vi "Color Manipulation.vi"() -> ()   [LabVIEW 2014]
doc: "Use this template to build a VI to use as a subVI."
uses:
  <vilib>/vision/NI_Vision_Development_Module.lvlib
panel:
  out "Dst":T1(plugin-control)
  out "Src":T1(plugin-control)
  # ":: MVi Framework V1.0 ::\nAuthor:Gaoke Yang\nEmail: gaoke.yang@yahoo.com\nWeb: www.mvicontrol.com\nCopyright (C) 2015, MVI Technologies All Rights Reserved"
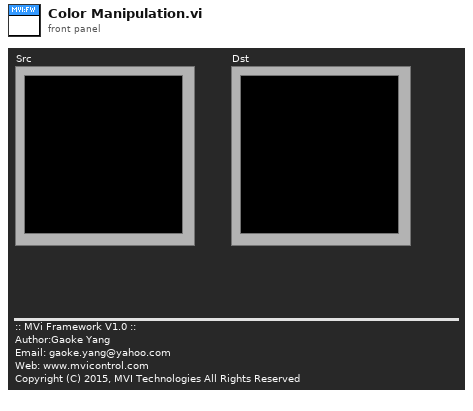
[diagram p1: front panel]
types:
  T1 = typedef "IMAQ Image.ctl" = refnum<image>
  T2 = typedef "Image Type" = u32
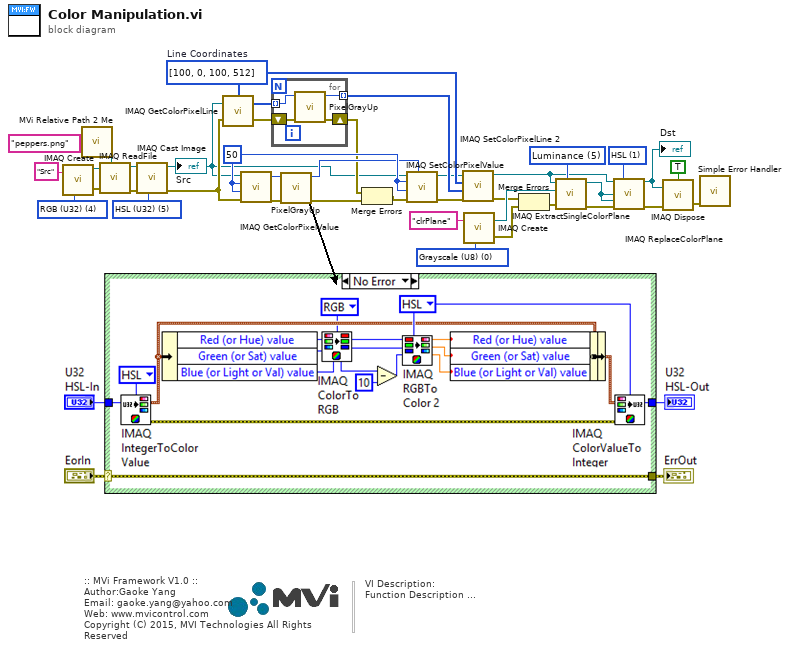
[diagram p0: block diagram]
diagram:
  w8 = u16 1 items=["RGB", "HSL", "HSV", "HSI"] ("Color Mode")
  w19 = 50 ("index")
  w21 = i32[] [100, 0, 100, 512]  # Line Coordinates
  w27 = T2 0 items=["Grayscale (U8)", "Grayscale (I16)", "Grayscale (SGL)", "Complex (CSG)", "RGB (U32)", "HSL (U32)", "RGB (U64)", "Grayscale (U16)"] ("Image Type")
  w28 = 5 items=["Red", "Green", "Blue", "Hue", "Saturation", "Luminance", "Value", "Intensity"] ("Color Plane")
  w29 = T2 4 items=["Grayscale (U8)", "Grayscale (I16)", "Grayscale (SGL)", "Complex (CSG)", "RGB (U32)", "HSL (U32)", "RGB (U64)", "Grayscale (U16)"] ("Image Type")
  w30 = T2 5 items=["Grayscale (U8)", "Grayscale (I16)", "Grayscale (SGL)", "Complex (CSG)", "RGB (U32)", "HSL (U32)", "RGB (U64)", "Grayscale (U16)"] ("Image Type")
  # "VI Description:\nFunction Description ..."
  # ":: MVi Framework V1.0 ::\nAuthor:Gaoke Yang\nEmail: gaoke.yang@yahoo.com\nWeb: www.mvicontrol.com\nCopyright (C) 2015, MVI Technologies All Rights Reserved"
  n1 = call "IMAQ Create"("Image Name"="Src" ("name or relative path"), "Image Type"=w29) -> ("New Image"=w34:T1, "error out"=w33:errorcluster)  [unwired: 2 in, 1 out]
  n2 = call "MVi Relative Path 2 Me.vi"("Relative Path"="peppers.png" ("name or relative path")) -> ("Appended Dir"=w35:path)  [unwired: 5 in, 1 out]
  n3 = call "IMAQ ReadFile"("File Path"=w35, "error in (no error)"=w33, "Image"=w34) -> ("error out"=w32:errorcluster, "Image Out"=w31:T1)  [unwired: 4 in, 3 out]
  n4 = call "IMAQ Cast Image"("Image Type"=w30, "error in (no error)"=w32, "Image Src"=w31) -> ("error out"=w9:errorcluster, "Image Dst Out"=w6:T1)  [unwired: 7 in]
  "Src" <- w6
  n5 = call "IMAQ GetColorPixelLine"("Line Coordinates"=w21, "Image"=w6, "error in (no error)"=w9) -> ("Pixels Line (U32)"=w24:u32[], "error out"=w23:errorcluster)  [unwired: 1 in, 1 out]
  n6 = call "IMAQ GetColorPixelValue"("error in (no error)"=w9, "Y Coordinate"=w19, "X Coordinate"=w19, "Image"=w6) -> ("error out"=w20:errorcluster, "Pixel Value (U32)"=w18:u32)  [unwired: 1 out]
  n7 = for {
    tunnel: w24 -> [w43] mode=indexing
    shift-right: [w41] -> w14
    shift-left: w23 -> [w42]
    tunnel: [w40] -> w22 mode=indexing
    n8 = call "PixelGrayUp.vi"("EorIn"=w42, "U32\nHSL-In"=w43) -> ("ErrOut"=w41:errorcluster, "U32\nHSL-Out"=w40:u32)  [unwired: 8 in]
  }
  n9 = call "PixelGrayUp.vi"("EorIn"=w20, "U32\nHSL-In"=w18) -> ("ErrOut"=w13:errorcluster, "U32\nHSL-Out"=w17:u32)  [unwired: 8 in]
  n10 = Merge Errors(w14, w13) -> (w12:errorcluster)
  n11 = call "IMAQ SetColorPixelValue"("Pixel Value (U32)"=w17, "error in (no error)"=w12, "Y Coordinate"=w19, "X Coordinate"=w19, "Image"=w6) -> ("error out"=w16:errorcluster, "Image Out"=w15:T1)  [unwired: 5 in]
  n12 = call "IMAQ SetColorPixelLine 2"("error in (no error)"=w16, "Pixels Line (U32)"=w22, "Line Coordinates"=w21, "Image"=w15) -> ("error out"=w5:errorcluster, "Image Out"=w3:T1)  [unwired: 6 in]
  n13 = call "IMAQ Create"("Image Name"="clrPlane" ("name or relative path"), "Image Type"=w27) -> ("New Image"=w25:T1, "error out"=w11:errorcluster)  [unwired: 2 in, 1 out]
  n14 = Merge Errors(w5, w11) -> (w10:errorcluster)
  n15 = call "IMAQ ExtractSingleColorPlane"("Color Plane"=w28, "error in (no error)"=w10, "Image Dst"=w25, "Image Src"=w3) -> ("error out"=w4:errorcluster, "Image Dst Out"=w1:T1)  [unwired: 6 in]
  n16 = call "IMAQ ReplaceColorPlane"("Image Src"=w3, "Color Mode"=w8, "Red or Hue Plane"=w1, "Green or Sat Plane"=w1, "error in (no error)"=w4) -> ("Image Dst Out"=w2:T1, "error out"=w7:errorcluster)  [unwired: 9 in]
  "Dst" <- w2
  n17 = call "IMAQ Dispose"("All Images? (No)"=TRUE, "Image"=w2, "error in (no error)"=w7) -> ("error out"=w36:errorcluster)  [unwired: 3 out]
  n18 = call <vilib>:"Simple Error Handler.vi"("error in (no error)"=w36) -> ()  [unwired: 1 in, 8 out]
